vi "Event Notification.Status Message.vi"(4 "Display":bool=TRUE, 5 "FWD":bool, 6 "Log":bool, 7 "Level":T1 caption="Level(Normal)", 9 "Message":string, 10 "Event Notification in":refnum<class "Event Notification.lvclass">) -> ()   [LabVIEW 2024, in "EQMF.lvlib" / "Event Log.lvlib" / "Event Notification.lvclass"]
uses:
  Event Notification.lvclass
  Event Log.Log Level.ctl
  Event Notification.lvclass/Event Notification.ctl
  Event Log.lvlib
  Queues/Queue Utils.lvlib
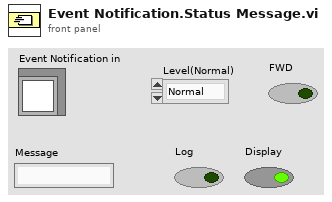
[diagram p1: front panel]
types:
  T1 = typedef "EQMF.lvlib/Event Log.lvlib/Event Log.Log Level.ctl" = enum16{"Normal", "Verbose", "Debug0", "Debug1", "Debug2"}
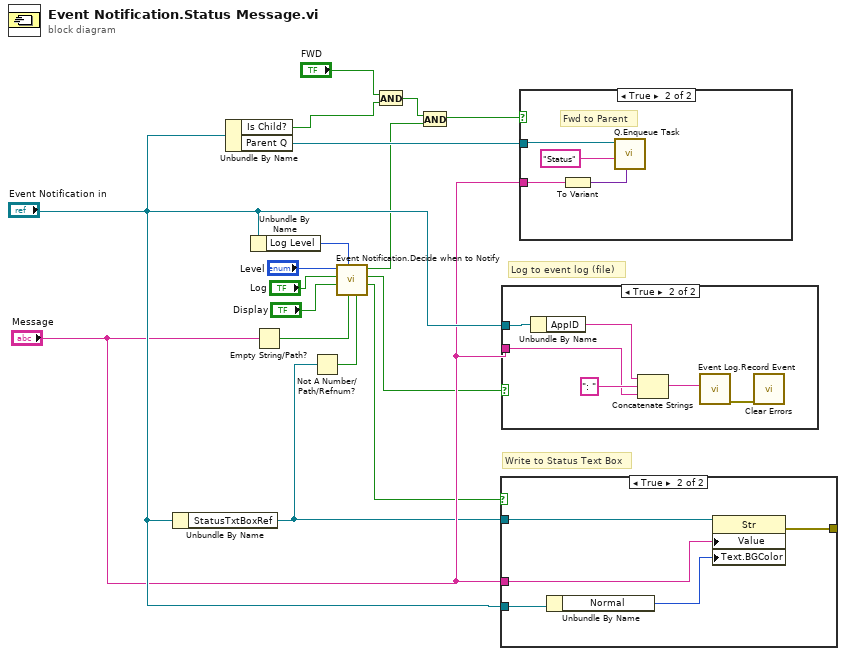
[diagram p0: block diagram]
diagram:
  # "Write to Status Text Box"
  # "Log to event log (file)"
  n1 = Unbundle By Name("Event Notification in") -> ("StatusTxtBoxRef"=w14:refnum<vi>)
  n2 = Unbundle By Name("Event Notification in") -> ("Is Child?"=w2:bool, "Parent Q"=w15:refnum<queue>)
  n3 = Unbundle By Name("Event Notification in") -> ("Log Level"=w13:T1)
  n4 = Empty String/Path?(string/path="Message") -> (empty?=w9:bool)
  n5 = Not A Number/Path/Refnum?(number/path/refnum=w14) -> (NaN/Path/Refnum?=w4:bool)
  n6 = call "Event Notification.Decide when to Notify.vi"("IsNotControlRef"=w4, "IsEmptyStr"=w9, "Sys Level"=w13, "Display"="Display", "Log"="Log", "Level"="Level") -> ("Display"=w5:bool, "Log"=w6:bool, "Fwd to Parent"=w7:bool)  [unwired: 3 in]
  n7 = And(x="FWD", y=w2) -> (x .and. y?=w1:bool)
  n8 = And(x=w1, y=w7) -> (x .and. y?=w8:bool)
  n9 = case shown="True" w5 {
    tunnel: "Message" -> [_ w20]
    tunnel: [_ w22] -> _
    tunnel: w14 -> [_ w21]
    tunnel: "Event Notification in" -> [_ w19]
    frame False {
    }
    frame True {
      n10 = Unbundle By Name(w19) -> ("Normal"=w18:u32)
      n11 = property class="Str"(reference=w21, "Value"=w20, "Text.BGColor"=w18) -> (error out=w22:errorcluster)  [unwired: 1 in, 1 out]
    }
  }
  n12 = case shown="True" w6 {
    tunnel: "Message" -> [_ w25]
    tunnel: "Event Notification in" -> [_ w28]
    frame False {
    }
    frame True {
      n13 = Unbundle By Name(w28) -> ("AppID"=w27:string)
      n14 = Concatenate Strings(w27, ": ", w25) -> (w24:string)
      n15 = call "Event Log.Record Event.vi"("Message"=w24) -> ("error out"=w23:errorcluster)  [unwired: 10 in]
      n16 = call <vilib>:"Clear Errors.vi"("error in (no error)"=w23) -> ()  [unwired: 5 in, 2 out]
    }
  }
  n17 = case shown="True" w8 {
    tunnel: w15 -> [_ w32]
    tunnel: "Message" -> [_ w29]
    frame False {
    }
    frame True {
      # "Fwd to Parent"
      n18 = To Variant(anything=w29) -> (Variant=w30:variant)
      n19 = call "Q.Enqueue Task.vi"("Data1"=w30, "Task Name"="Status", "Q In"=w32) -> ()  [unwired: 7 in, 2 out]
    }
  }
